vi "get VTK Data.vi"(8 "error in (no error)":errorcluster, 11 "vtkdata 2":dbl[][](array[numeric])) -> (0 "error out":errorcluster, 3 "vtkdata 3":dbl[][](array[numeric]))   [LabVIEW 2019, in "libConvectionDiffusionWrapper.lvlib"]
doc: "void getVTK_Data(double (&vtkdata)[100][100]);"
uses:
  libConvectionDiffusionWrapper.lvlib
  libConvectionDiffusionWrapper.so
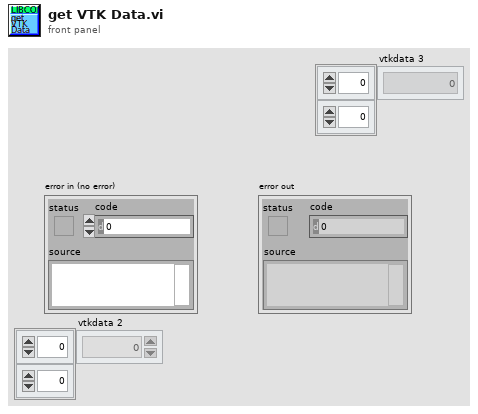
[diagram p1: front panel]
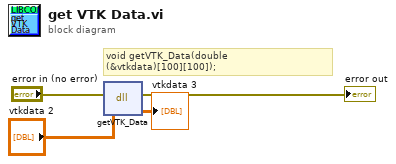
[diagram p0: block diagram]
diagram:
  # "void getVTK_Data(double (&vtkdata)[100][100]);"
  n1 = dll-call lib="home/paul/Schreibtisch/Convection_diffusion/LabView/lib/libConvectionDiffusionWrapper.*" fn="getVTK_Data"(error in="error in (no error)", "vtkdata"="vtkdata 2") -> (error out=→"error out":errorcluster, "vtkdata"=→"vtkdata 3":dbl[][])  [unwired: 3 in, 1 out]
